vi "Untitled 0.vi"() -> ()   [LabVIEW 2021]
panel:
  out "Waveform Graph 3":dynamicdata(graph)
  out "Waveform Graph 2":dynamicdata(graph)
  out "Waveform Graph":dynamicdata(graph)
  in  "Boolean":bool
  in  "name or relative path 2":path=path "../1.tdms"
  in  "stop (F)":bool
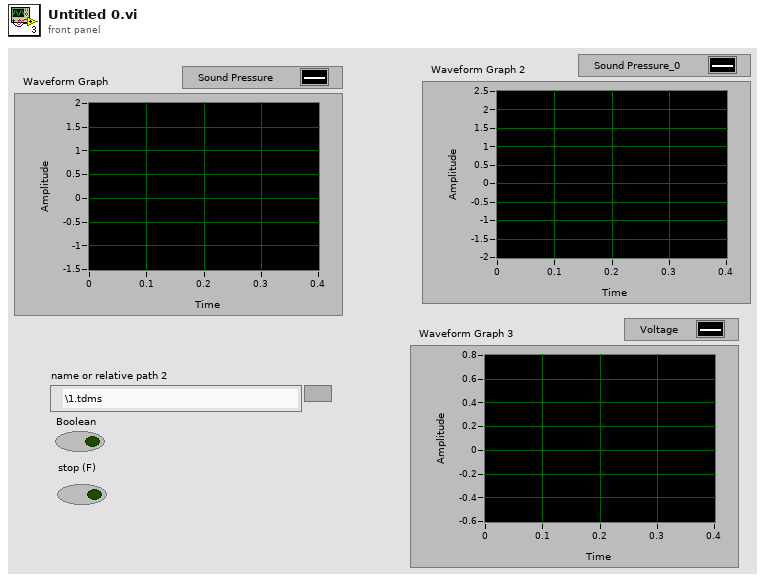
[diagram p1: front panel]
types:
  T1 = enum16{"open", "open or create", "create or replace", "create", "open (read-only)"}
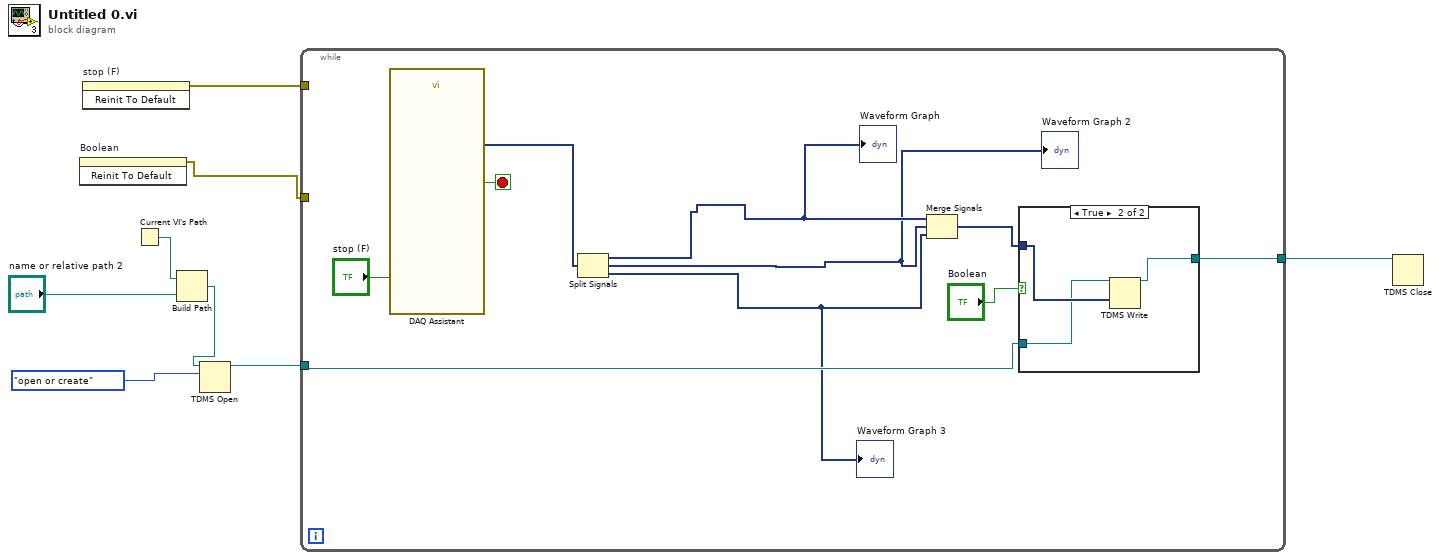
[diagram p0: block diagram]
diagram:
  n1 = invoke on="Boolean" class="Bool (strict)" method="Reinit To Default"() -> (error out=w3:errorcluster)  [unwired: 3 in, 2 out]
  n2 = invoke on="stop (F)" class="Bool (strict)" method="Reinit To Default"() -> (error out=w1:errorcluster)  [unwired: 3 in, 2 out]
  n3 = Current VI's Path() -> (path=w8:path)
  n4 = Build Path(base path=w8, name or relative path="name or relative path 2") -> (appended path=w7:path)
  n5 = TDMS Open(10:T1."open or create" ("operation (0:open)"), 11:w7) -> (3:w2:refnum<k34>)  [unwired: 5 in, 1 out]
  n6 = while {
    tunnel: [w13] -> w4
    tunnel: w3 -> [_]
    tunnel: w2 -> [w12]
    tunnel: w1 -> [_]
    stop <- w17 stop-if-true
    n7 = call "DAQ Assistant"("stop (F)"="stop (F)") -> ("data"=w16:dynamicdata, "stopped"=w17:bool)  [unwired: 15 in, 2 out]
    n8 = Split Signals(w16) -> (w10:dynamicdata, w9:dynamicdata, w11:dynamicdata)  [unwired: 3 in]
    "Waveform Graph" <- w10
    "Waveform Graph 2" <- w9
    "Waveform Graph 3" <- w11
    n9 = Merge Signals(w10, w9, w11) -> (w14:dynamicdata)
    n10 = case shown="True" "Boolean" {
      tunnel: w14 -> [_ w22]
      tunnel: [w19 w21] -> w13
      tunnel: w12 -> [w19 w20]
      frame False {
      }
      frame True {
        n11 = TDMS Write(0:w20, 9:w22) -> (4:w21:refnum<k34>)  [unwired: 4 in, 3 out]
      }
    }
  }
  n12 = TDMS Close(11:w4) -> ()  [unwired: 1 in, 2 out]
